vi "Position in Top Right.vi"(8 "error in (no error)":errorcluster, 11 "Width of Control (%)":dbl) -> (0 "error out":errorcluster, 3 "Right Pos":u32)   [LabVIEW 2014]
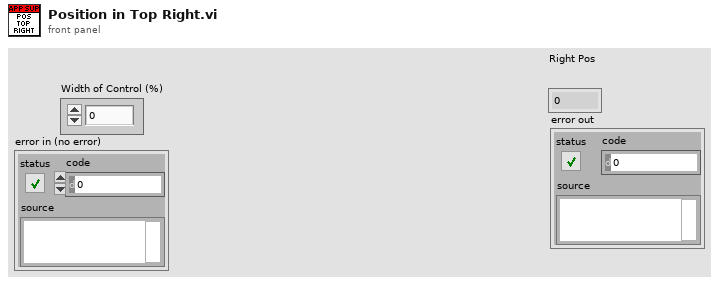
[diagram p1: front panel]
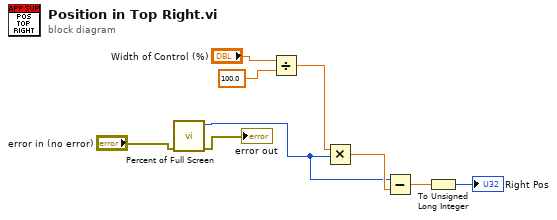
[diagram p0: block diagram]
diagram:
  n1 = call "Percent of Full Screen.vi"("error in (no error)"="error in (no error)") -> ("error out"=→"error out":errorcluster, "Right"=w1:i16)  [unwired: 8 in, 1 out]
  n2 = Divide(x="Width of Control (%)", y=100.0) -> (x/y=w7:dbl)
  n3 = Multiply(x=w7, y=w1) -> (x*y=w6:dbl)
  n4 = Subtract(x=w1, y=w6) -> (x-y=w5:dbl)
  n5 = To Unsigned Long Integer(number=w5) -> (unsigned 32bit integer=→"Right Pos":u32)
